vi "subvi_ByteArrayToPaddedByteArray.vi"(6 "Padding Mask In":bool[](array[boolean]), 7 "#pragma directive (0, default)":i32, 8 "error in (no error)":errorcluster, 9 "Element Sizes":i32[](array[numeric]), 10 "Alignment Targets":i32[](array[numeric]), 11 "Cluster Data as Byte Array":u8[](array[numeric])) -> (0 "error out":errorcluster, 1 "Total Size":i32, 2 "Alignment Target Out":i32, 3 "Bytes Out (Padded as Needed)":u8[](array[numeric])=[0, 0, 0, 0, 204, 204, 204, 204, 64, 129, 88, 0, 0, 0, 0, 0, 0, 0, 0, 0, 0, 0, 0, 0, 0, 0, 0, 0, 0, 0, 0, 0, 0, 0, 0, 0, 0, 0, 0, 0, 255, 255, 255, 255, 0, 0, 0, 0, 0, 0, 0, 0, 0, 0, 0, 0, 0, 0, 0, 0, 0, 0, 0, 0, 0, 0, 0, 0, 0, 0, 0, 0, 0, 0, 0, 0, 0, 0, 0, 0, 0, 0, 0, 0, 0, 0, 0, 0, 3, 79, 181, 227, 0, 0, 0, 44, 0, 0, 0, 0, 0, 0, 0, 0, 0, 0, 0, 0, 0, 0, 0, 0, 0, 0, 0, 0, 0, 0, 0, 0, 0, 0, 0, 0, 0, 0, 0, 0, 0, 0, 0, 44, 204, 204, 204, 204, 0, 0, 0, 0, 0, 0, 0, 0, 64, 254, 15, 48, 0, 0, 0, 0, 0, 0, 0, 0, 0, 0, 0, 0, 0, 0, 0, 0, 0, 0, 0, 0, 0, 0, 0, 0, 0, 0, 0, 123], 4 "Padding Mask Out":bool[](array[boolean]), 5 "Size without padding":i32)   [LabVIEW 2020]
doc: "Takes byte array and underlying element \"sizes\" and evaluates each element alignment against packing rules. Rules vary by #pragma packing directive, data types included in the struct, as well as last element/whole structure evaluation."
panel:
  # "### BSD License (http://www.opensource.org/licenses/bsd-license.php) Begin ###\n \nCopyright (c) 2014 Jeffrey Holt <jolt.holt@gmail.com>\n\nAll rights reserved.\n\nRedistribution and use in source and binary forms, with or without modification, are permitted provided that the following conditions are met:\n\n    * Redistributions of source code must retain the above copyright notice\n\nTHIS SOFTWARE IS PROVIDED BY THE COPYRIGHT HOLDERS AND CONTRIBUTORS \"AS IS\" AND ANY EXPRESS OR IMPLIED WARRANTIES, \nINCLUDING, BUT NOT LIMITED TO, THE IMPLIED WARRANTIES OF MERCHANTABILITY AND FITNESS FOR A PARTICULAR PURPOSE ARE \nDISCLAIMED. IN NO EVENT SHALL THE COPYRIGHT OWNER OR CONTRIBUTORS BE LIABLE FOR ANY DIRECT, INDIRECT, INCIDENTAL,\n SPECIAL, EXEMPLARY, OR CONSEQUENTIAL DAMAGES (INCLUDING, BUT NOT LIMITED TO, PROCUREMENT OF SUBSTITUTE GOODS OR \nSERVICES; LOSS OF USE, DATA, OR PROFITS; OR BUSINESS INTERRUPTION) HOWEVER CAUSED AND ON ANY THEORY OF LIABILITY, \nWHETHER IN CONTRACT, STRICT LIABILITY, OR TORT (INCLUDING NEGLIGENCE OR OTHERWISE) ARISING IN ANY WAY OUT OF THE USE \nOF THIS SOFTWARE, EVEN IF ADVISED OF THE POSSIBILITY OF SUCH DAMAGE.\n\n### BSD License End ###"
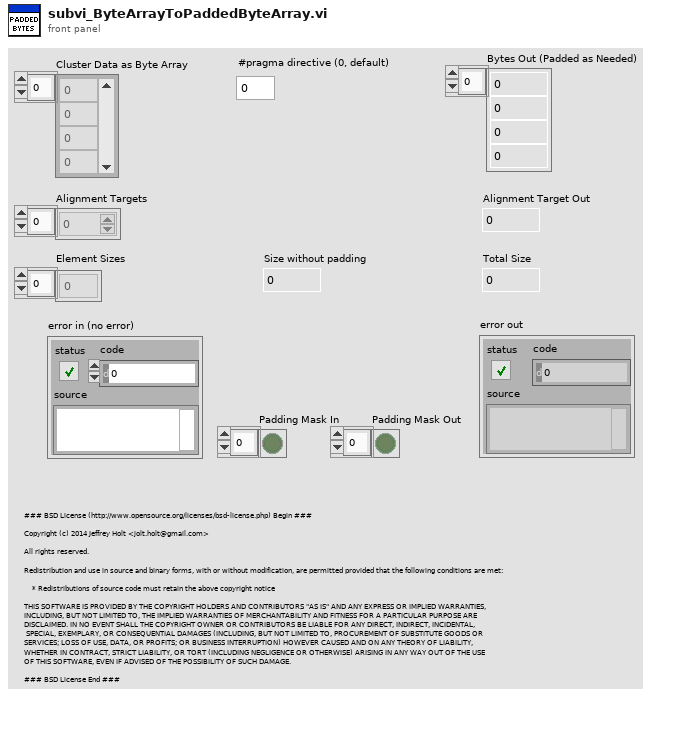
[diagram p1: front panel]
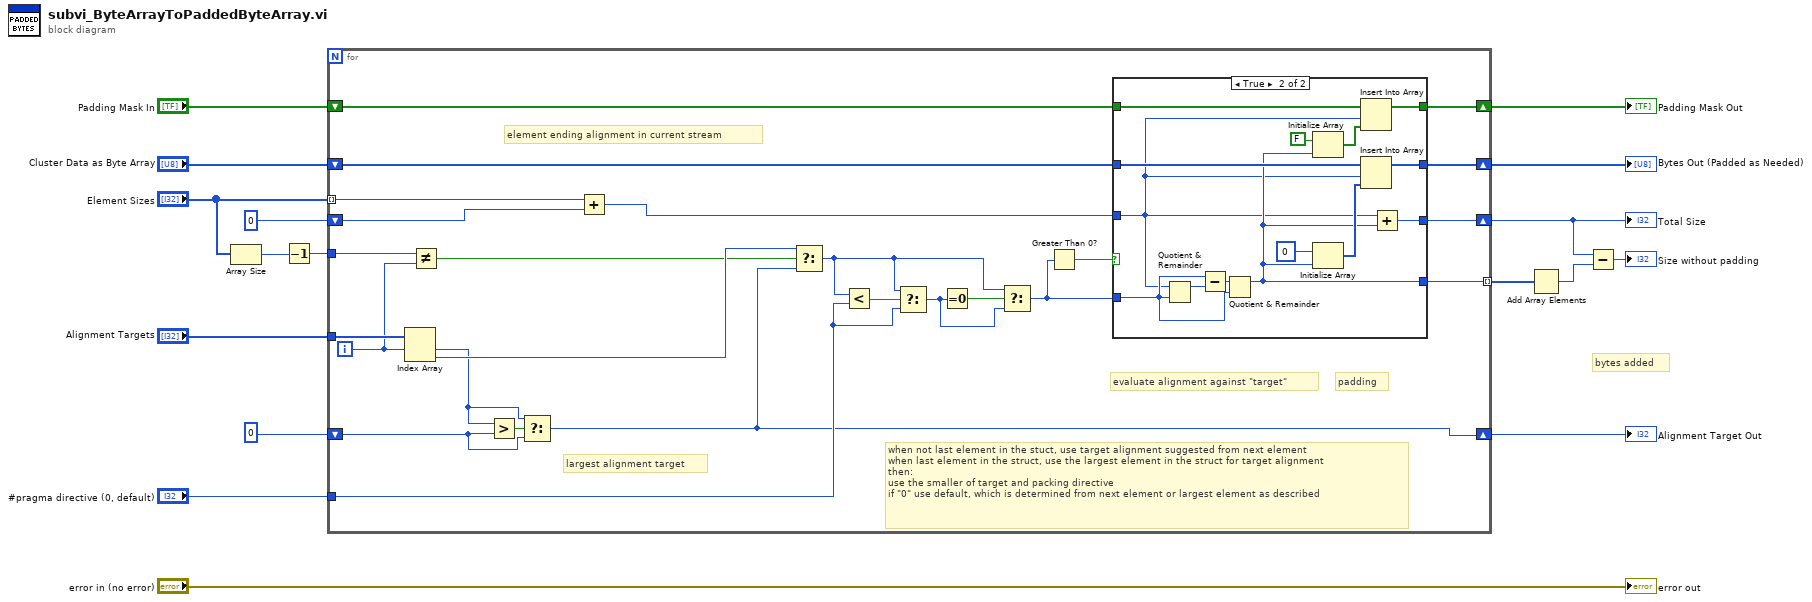
[diagram p0: block diagram]
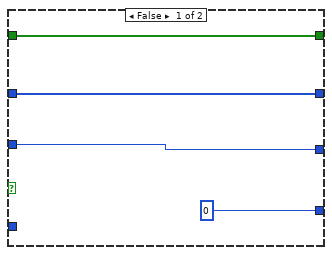
[diagram p2: hidden frame]
diagram:
  # "bytes added"
  n1 = Array Size(array="Element Sizes") -> (size(s)=w15:i32)
  n2 = Decrement(x=w15) -> (x-1=w14:i32)
  n3 = for {
    tunnel: "Alignment Targets" -> [w42]
    shift-right: [w21] -> w10
    shift-left: 0 -> [w41]
    shift-right: [w18] -> w8
    shift-left: 0 -> [w39]
    tunnel: w14 -> [w37]
    tunnel: "#pragma directive (0, default)" -> [w36]
    tunnel: [w23] -> w11 mode=indexing
    tunnel: "Element Sizes" -> [w28] mode=indexing
    shift-right: [w24] -> w5
    shift-left: "Cluster Data as Byte Array" -> [w25]
    shift-right: [w19] -> w2
    shift-left: "Padding Mask In" -> [w20]
    i -> [w38]
    # "element ending alignment in current stream"
    # "evaluate alignment against \"target\""
    # "padding"
    # "when not last element in the stuct, use target alignment suggested from next element\nwhen last element in the struct, use the largest element in the struct for target alignment\nthen:\nuse the smaller of target and packing directive\nif \"0\" use default, which is determined from next element or largest element as described"
    # "largest alignment target"
    n4 = Index Array(array=w42, index #1=w38) -> (element #1=w29:i32, element #2=w31:i32)  [unwired: 1 in]
    n5 = Not Equal?(x=w37, y=w38) -> (x != y?=w30:bool)
    n6 = Greater?(x=w29, y=w39) -> (0:w40:bool)
    n7 = Select(t=w29, s=w40, f=w39) -> (s? t:f=w18:i32)
    n8 = Add(x=w28, y=w41) -> (x+y=w22:i32)
    n9 = Select(t=w31, s=w30, f=w18) -> (s? t:f=w32:i32)
    n10 = Less?(x=w32, y=w36) -> (x < y?=w35:bool)
    n11 = Select(t=w32, s=w35, f=w36) -> (s? t:f=w33:i32)
    n12 = Equal To 0?(x=w33) -> (x = 0?=w34:bool)
    n13 = Select(t=w32, s=w34, f=w33) -> (s? t:f=w26:i32)
    n14 = Greater Than 0?(x=w26) -> (x > 0?=w27:bool)
    n15 = case shown="True" w27 {
      tunnel: [w46 w60] -> w24
      tunnel: [0 w51] -> w23
      tunnel: w25 -> [w46 w54]
      tunnel: w26 -> [_ w56]
      tunnel: w22 -> [w44 w48]
      tunnel: [w44 w53] -> w21
      tunnel: w20 -> [w43 w52]
      tunnel: [w43 w47] -> w19
      frame False {
      }
      frame True {
        n16 = Quotient & Remainder(x=w48, y=w56) -> (x-y*floor(x/y)=w57:i32)  [unwired: 1 out]
        n17 = Subtract(x=w56, y=w57) -> (x-y=w58:i32)
        n18 = Quotient & Remainder(x=w58, y=w56) -> (x-y*floor(x/y)=w51:i32)  [unwired: 1 out]
        n19 = Initialize Array(FALSE, w51) -> (w49:bool[])
        n20 = Initialize Array(u8 0, w51) -> (w55:u8[])
        n21 = Insert Into Array(array=w52, index=w48, new element=w49) -> (w47:bool[])
        n22 = Insert Into Array(array=w54, index=w48, new element=w55) -> (w60:u8[])
        n23 = Add(x=w48, y=w51) -> (x+y=w53:i32)
      }
    }
  }
  "Bytes Out (Padded as Needed)" <- w5
  "Total Size" <- w10
  "Alignment Target Out" <- w8
  "Padding Mask Out" <- w2
  n24 = Add Array Elements(numeric array=w11) -> (sum=w1:i32)
  n25 = Subtract(x=w10, y=w1) -> (x-y=→"Size without padding":i32)
  "error out" <- "error in (no error)"
